vi "Fetch Single Measurement (Current).vi"(0 "VISA resource name":refnum<visa-resource-name>, 11 "error in (no error)":errorcluster) -> (3 "Peak Current":dbl, 4 "VISA resource name out":refnum<visa-resource-name>, 6 "DC Current":dbl, 8 "AC RMS Current":dbl, 10 "AC + DC RMS Current":dbl, 15 "error out":errorcluster)   [LabVIEW 2020, in "Agilent 681x Series.lvlib"]
doc: "Fetches and returns instantaneous current measurements.\n\n<B>Note:</B>\n\nUse this VI only with other low-level VIs. The high-level VIs automatically incorporate this functionality. This VI does not check the instrument status. If you want to check the instrument status, call the Error Query VI at the conclusion of the sequence."
uses:
  <instrlib>/Agilent 681x Series/Agilent 681x Series.lvlib
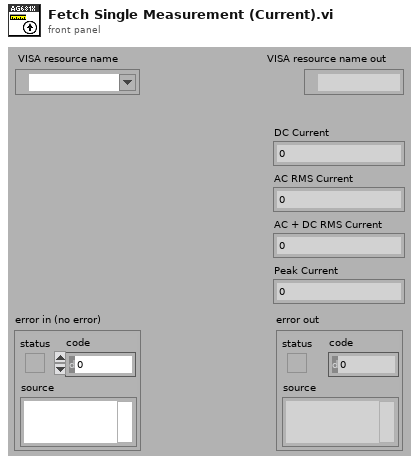
[diagram p1: front panel]
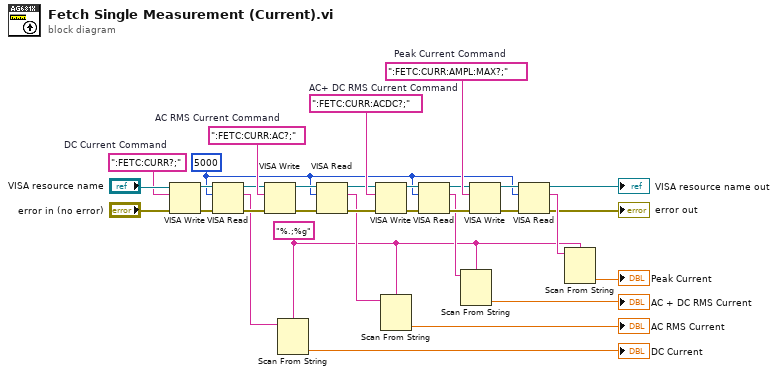
[diagram p0: block diagram]
diagram:
  w5 = "%.;%g"
  w18 = ":FETC:CURR:AMPL:MAX?;"  # Peak Current Command
  w19 = ":FETC:CURR:ACDC?;"  # AC+ DC RMS Current Command
  w27 = ":FETC:CURR:AC?;"  # AC RMS Current Command
  w13 = u32 5000 ("byte count")
  w28 = ":FETC:CURR?;"  # DC Current Command
  n1 = VISA Write(VISA resource name="VISA resource name", write buffer=w28, error in (no error)="error in (no error)") -> (VISA resource name out=w29:refnum<visa-resource-name>, error out=w30:errorcluster)  [unwired: 1 out]
  n2 = VISA Read(VISA resource name=w29, byte count=w13, error in (no error)=w30) -> (VISA resource name out=w21:refnum<visa-resource-name>, read buffer=w11:string, error out=w20:errorcluster)  [unwired: 1 out]
  n3 = VISA Write(VISA resource name=w21, write buffer=w27, error in (no error)=w20) -> (VISA resource name out=w26:refnum<visa-resource-name>, error out=w12:errorcluster)  [unwired: 1 out]
  n4 = Scan From String(format string=w5, input string=w11) -> (output 1=→"DC Current":dbl)  [unwired: 3 in, 3 out]
  n5 = VISA Read(VISA resource name=w26, byte count=w13, error in (no error)=w12) -> (VISA resource name out=w14:refnum<visa-resource-name>, read buffer=w10:string, error out=w15:errorcluster)  [unwired: 1 out]
  n6 = VISA Write(VISA resource name=w14, write buffer=w19, error in (no error)=w15) -> (VISA resource name out=w24:refnum<visa-resource-name>, error out=w25:errorcluster)  [unwired: 1 out]
  n7 = Scan From String(format string=w5, input string=w10) -> (output 1=→"AC RMS Current":dbl)  [unwired: 3 in, 3 out]
  n8 = VISA Read(VISA resource name=w24, byte count=w13, error in (no error)=w25) -> (VISA resource name out=w17:refnum<visa-resource-name>, read buffer=w9:string, error out=w16:errorcluster)  [unwired: 1 out]
  n9 = Scan From String(format string=w5, input string=w9) -> (output 1=→"AC + DC RMS Current":dbl)  [unwired: 3 in, 3 out]
  n10 = VISA Write(VISA resource name=w17, write buffer=w18, error in (no error)=w16) -> (VISA resource name out=w23:refnum<visa-resource-name>, error out=w22:errorcluster)  [unwired: 1 out]
  n11 = VISA Read(VISA resource name=w23, byte count=w13, error in (no error)=w22) -> (VISA resource name out=→"VISA resource name out":refnum<visa-resource-name>, read buffer=w8:string, error out=→"error out":errorcluster)  [unwired: 1 out]
  n12 = Scan From String(format string=w5, input string=w8) -> (output 1=→"Peak Current":dbl)  [unwired: 3 in, 3 out]
